vi "UpdateFieldVars.vi"(8 "error in (no error)":errorcluster) -> (0 "error out":errorcluster)   [LabVIEW 2015]
uses:
  Classes/MotorControl/TypeDef/ControllerMode.ctl
  Classes/MotorControl/MotorControl.lvclass
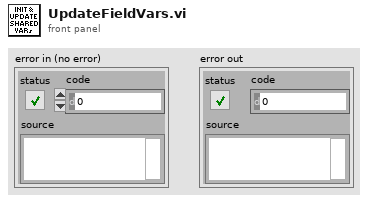
[diagram p1: front panel]
types:
  T1 = typedef "MotorControl.lvclass/ControllerMode.ctl" = enum16{"Idle", "FF", "PID"}
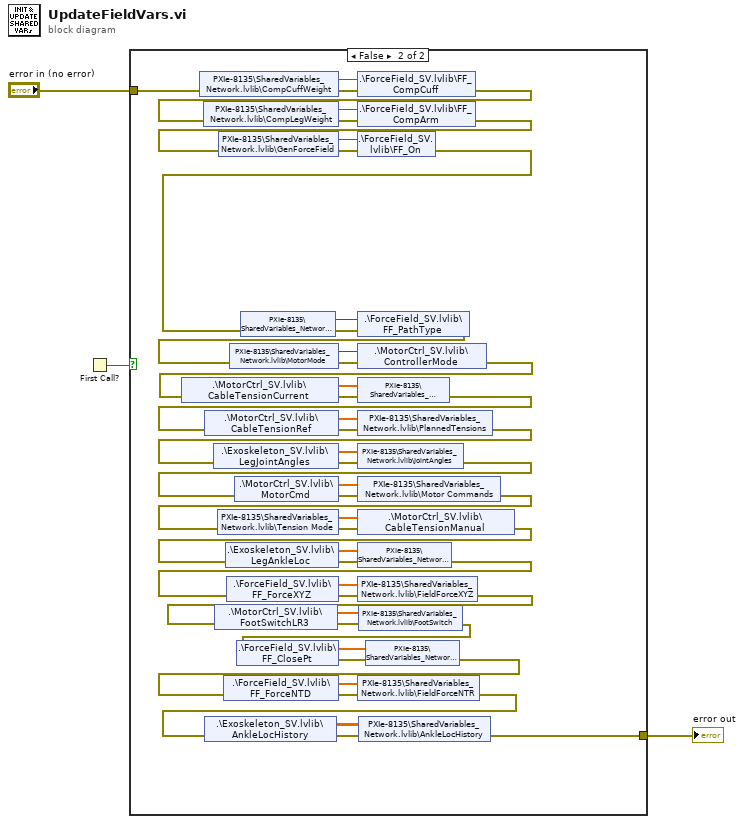
[diagram p0: block diagram]
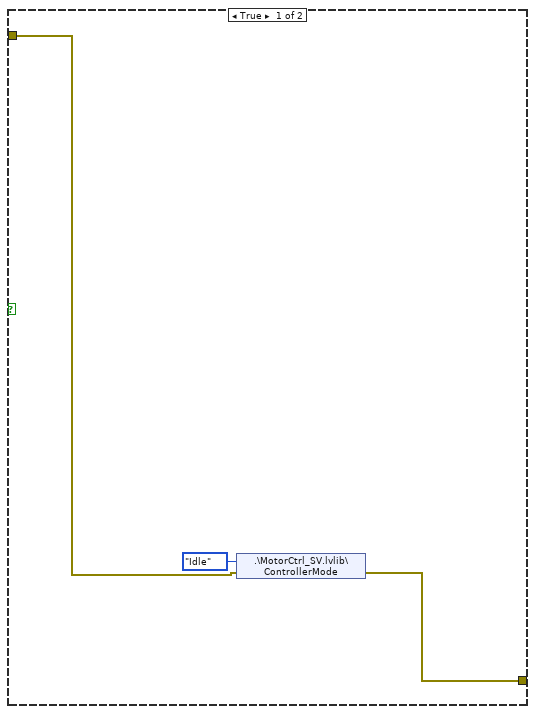
[diagram p2: hidden frame]
diagram:
  n1 = First Call?() -> (First Call?: T/F=w1:bool)
  n2 = case shown="False" w1 {
    tunnel: [w6 w8] -> w3
    tunnel: "error in (no error)" -> [w4 w19]
    frame True {
      n3 = shared-variable ".\\MotorCtrl_SV.lvlib\\ControllerMode"(ControllerMode."Idle" ("MoterMode"), error in=w4) -> (error out=w6:errorcluster)
    }
    frame False {
      n4 = shared-variable "PXIe-8135\\SharedVariables_Network.lvlib\\CompCuffWeight"(error in=w19) -> (w27:bool, error out=w26:errorcluster)
      n5 = shared-variable ".\\ForceField_SV.lvlib\\FF_CompCuff"(w27, error in=w26) -> (error out=w20:errorcluster)
      n6 = shared-variable "PXIe-8135\\SharedVariables_Network.lvlib\\CompLegWeight"(error in=w20) -> (w25:bool, error out=w24:errorcluster)
      n7 = shared-variable ".\\ForceField_SV.lvlib\\FF_CompArm"(w25, error in=w24) -> (error out=w21:errorcluster)
      n8 = shared-variable "PXIe-8135\\SharedVariables_Network.lvlib\\GenForceField"(error in=w21) -> (w23:bool, error out=w22:errorcluster)
      n9 = shared-variable ".\\ForceField_SV.lvlib\\FF_On"(w23, error in=w22) -> (error out=w7:errorcluster)
      n10 = shared-variable "PXIe-8135\\SharedVariables_Network.lvlib\\PathType"(error in=w7) -> (w31:u8, error out=w30:errorcluster)
      n11 = shared-variable ".\\ForceField_SV.lvlib\\FF_PathType"(w31, error in=w30) -> (error out=w29:errorcluster)
      n12 = shared-variable "PXIe-8135\\SharedVariables_Network.lvlib\\MotorMode"(error in=w29) -> (w35:T1, error out=w34:errorcluster)
      n13 = shared-variable ".\\MotorCtrl_SV.lvlib\\ControllerMode"(w35, error in=w34) -> (error out=w28:errorcluster)
      n14 = shared-variable ".\\MotorCtrl_SV.lvlib\\CableTensionCurrent"(error in=w28) -> (w36:dbl[], error out=w37:errorcluster)
      n15 = shared-variable "PXIe-8135\\SharedVariables_Network.lvlib\\Tensions"(w36, error in=w37) -> (error out=w48:errorcluster)
      n16 = shared-variable ".\\MotorCtrl_SV.lvlib\\CableTensionRef"(error in=w48) -> (w38:dbl[], error out=w39:errorcluster)
      n17 = shared-variable "PXIe-8135\\SharedVariables_Network.lvlib\\PlannedTensions"(w38, error in=w39) -> (error out=w49:errorcluster)
      n18 = shared-variable ".\\Exoskeleton_SV.lvlib\\LegJointAngles"(error in=w49) -> (w41:dbl[], error out=w40:errorcluster)
      n19 = shared-variable "PXIe-8135\\SharedVariables_Network.lvlib\\JointAngles"(w41, error in=w40) -> (error out=w50:errorcluster)
      n20 = shared-variable ".\\MotorCtrl_SV.lvlib\\MotorCmd"(error in=w50) -> (w42:dbl[], error out=w43:errorcluster)
      n21 = shared-variable "PXIe-8135\\SharedVariables_Network.lvlib\\Motor Commands"(w42, error in=w43) -> (error out=w51:errorcluster)
      n22 = shared-variable "PXIe-8135\\SharedVariables_Network.lvlib\\Tension Mode"(error in=w51) -> (w44:dbl[], error out=w45:errorcluster)
      n23 = shared-variable ".\\MotorCtrl_SV.lvlib\\CableTensionManual"(w44, error in=w45) -> (error out=w52:errorcluster)
      n24 = shared-variable ".\\Exoskeleton_SV.lvlib\\LegAnkleLoc"(error in=w52) -> (w46:dbl[], error out=w47:errorcluster)
      n25 = shared-variable "PXIe-8135\\SharedVariables_Network.lvlib\\AnklePos"(w46, error in=w47) -> (error out=w55:errorcluster)
      n26 = shared-variable ".\\ForceField_SV.lvlib\\FF_ForceXYZ"(error in=w55) -> (w53:dbl[], error out=w54:errorcluster)
      n27 = shared-variable "PXIe-8135\\SharedVariables_Network.lvlib\\FieldForceXYZ"(w53, error in=w54) -> (error out=w15:errorcluster)
      n28 = shared-variable ".\\MotorCtrl_SV.lvlib\\FootSwitchLR3"(error in=w15) -> (w14:dbl[], error out=w13:errorcluster)
      n29 = shared-variable "PXIe-8135\\SharedVariables_Network.lvlib\\FootSwitch"(w14, error in=w13) -> (error out=w12:errorcluster)
      n30 = shared-variable ".\\ForceField_SV.lvlib\\FF_ClosePt"(error in=w12) -> (w18:dbl[], error out=w17:errorcluster)
      n31 = shared-variable "PXIe-8135\\SharedVariables_Network.lvlib\\ClosestPt"(w18, error in=w17) -> (error out=w16:errorcluster)
      n32 = shared-variable ".\\ForceField_SV.lvlib\\FF_ForceNTD"(error in=w16) -> (w33:dbl[], error out=w32:errorcluster)
      n33 = shared-variable "PXIe-8135\\SharedVariables_Network.lvlib\\FieldForceNTR"(w33, error in=w32) -> (error out=w11:errorcluster)
      n34 = shared-variable ".\\Exoskeleton_SV.lvlib\\AnkleLocHistory"(error in=w11) -> (w10:dbl[][], error out=w9:errorcluster)
      n35 = shared-variable "PXIe-8135\\SharedVariables_Network.lvlib\\AnkleLocHistory"(w10, error in=w9) -> (error out=w8:errorcluster)
    }
  }
  "error out" <- w3
